vi "Debug.vi"(8 "error in (no error)":errorcluster, 11 "cRIO Vacuum in":refnum<class "cRIO Vacuum.lvclass">) -> (0 "error out":errorcluster, 3 "cRIO Vacuum out":refnum<class "cRIO Vacuum.lvclass">)   [LabVIEW 2015, in "cRIO-Carbondioxide.lvlib" / "CO2-Actor.lvlib" / "cRIO Vacuum.lvclass"]
uses:
  cRIO Vacuum.lvclass
  cRIO Vacuum.lvclass/cRIO Vacuum.ctl
  CO2 Actor/CO2 Actor.lvclass
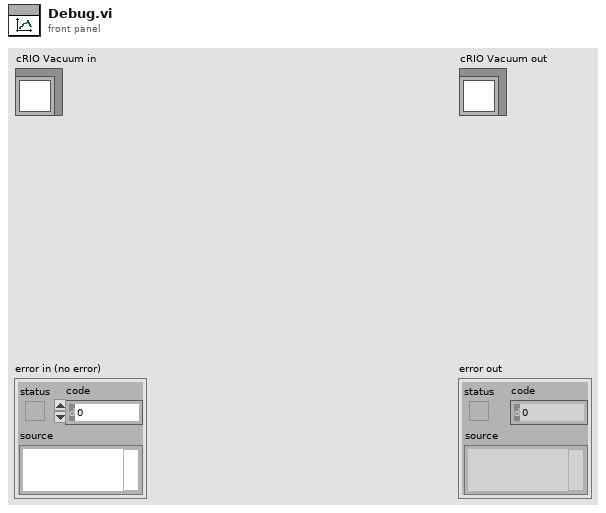
[diagram p1: front panel]
types:
  T1 = cluster{"Numeric 1":dbl, "Numeric 2":dbl, "Numeric 3":dbl, "Numeric 4":dbl, "Numeric 5":dbl, "Numeric 6":dbl, "Numeric 7":dbl, "Numeric 8":dbl}
  T2 = typedef "cRIO-Carbondioxide.lvlib/cRIO-CO2.lvlib/cRIO-CO2.lvclass/Debugger.ctl" = cluster{"Log Ref":refnum<vi>, "Debugger Graph Chart Ref":refnum<vi>, "Debug Rng Ref":refnum<vi>}
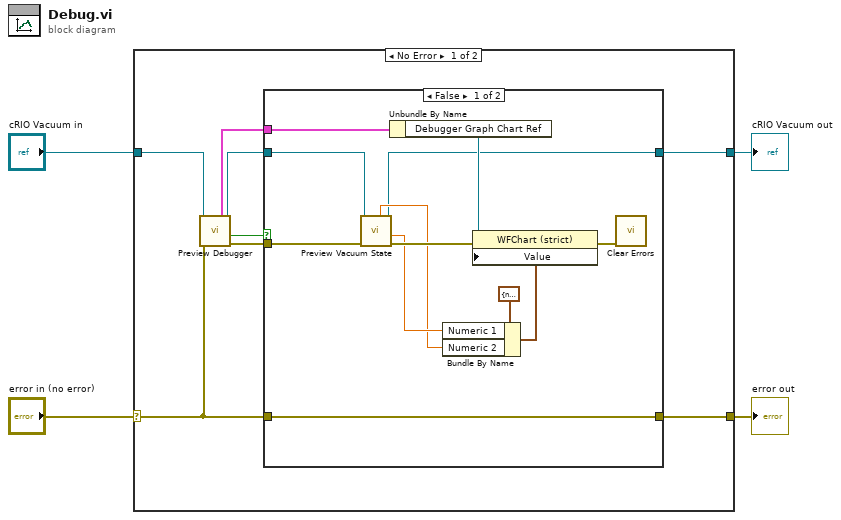
[diagram p0: block diagram]
diagram:
  n1 = case shown="No Error" "error in (no error)" {
    selector: "error in (no error)" -> [w5 w28]
    tunnel: [w6 w28] -> w3
    tunnel: [w8 w27] -> w1
    tunnel: "cRIO Vacuum in" -> [w11 w27]
    frame No Error {
      n2 = call "Preview Debugger.vi"("error in (no error)"=w5, "CO2 Actor in"=w11) -> ("error out"=w12:errorcluster, "timed out?"=w10:bool, "Debugger"=w9:T2, "CO2 Actor out"=w7:refnum<class "cRIO Vacuum.lvclass">)  [unwired: 6 in]
      n3 = case shown="False" w10 {
        tunnel: w12 -> [w14 _]
        tunnel: w9 -> [w21 _]
        tunnel: [w15 w26] -> w8
        tunnel: w7 -> [w13 w26]
        tunnel: [w19 w25] -> w6
        tunnel: w5 -> [w19 w25]
        frame False {
          n4 = call "Preview Vacuum State.vi"("error in (no error)"=w14, "cRIO Vacuum in"=w13) -> ("error out"=w18:errorcluster, "Pressure (mBar)"=w17:dbl, "cRIO Vacuum out"=w15:refnum<class "cRIO Vacuum.lvclass">, "d/dt"=w16:dbl)  [unwired: 3 in, 3 out]
          n5 = Unbundle By Name(w21) -> ("Debugger Graph Chart Ref"=w20:refnum<vi>)
          n6 = Bundle By Name(cluster=T1 {"Numeric 1"=nan, "Numeric 2"=nan, "Numeric 3"=nan, "Numeric 4"=nan, "Numeric 5"=nan, "Numeric 6"=nan, "Numeric 7"=nan, "Numeric 8"=nan} ("Cluster"), "Numeric 1"=w17, "Numeric 2"=w16) -> (w22:T1)
          n7 = property class="WFChart (strict)"(reference=w20, error in=w18, "Value"=w22) -> (error out=w24:errorcluster)  [unwired: 1 out]
          n8 = call <vilib>:"Clear Errors.vi"("error in (no error)"=w24) -> ()  [unwired: 5 in, 2 out]
        }
        frame True {
        }
      }
    }
    frame Error {
    }
  }
  "error out" <- w3
  "cRIO Vacuum out" <- w1
